vi "configwrite_ini.vi"() -> ()   [LabVIEW 2013]
uses:
  <vilib>/Utility/config.llb/Write Key (Double).vi
  <vilib>/Utility/config.llb/Write Key (String).vi
  <vilib>/Utility/config.llb/NI_LVConfig.lvlib
panel:
  out "error out":errorcluster caption="错误输出"
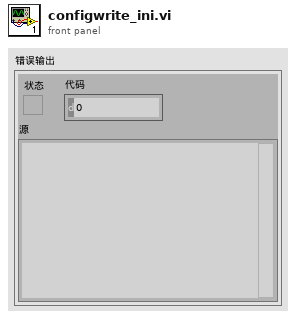
[diagram p1: front panel]
types:
  T1 = typedef "NI_LVConfig.lvlib/Config Data RefNum.ctl" = refnum<k1>
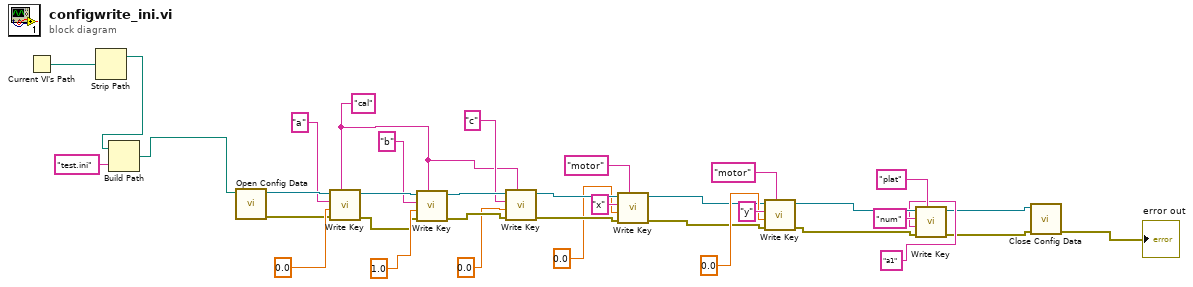
[diagram p0: block diagram]
diagram:
  w22 = "cal" ("section")
  n1 = Current VI's Path() -> (path=w2:path)
  n2 = Strip Path(path=w2) -> (stripped path=w1:path)  [unwired: 1 out]
  n3 = Build Path(base path=w1, name or relative path="test.ini" ("名称或相对路径")) -> (appended path=w3:path)
  n4 = call <vilib>:"Open Config Data.vi"("configuration file path"=w3) -> ("error out"=w27:errorcluster, "refnum"=w34:T1)  [unwired: 8 in, 1 out]
  n5 = call-poly <vilib>:"Write Key.vi"("section"=w22, "error in (no error)"=w27, "value"=0.0, "key"="a", "refnum"=w34) -> ("error out"=w28:errorcluster, "refnum out"=w31:T1)  [unwired: 4 in, 1 out]
  n6 = call-poly <vilib>:"Write Key.vi"("section"=w22, "error in (no error)"=w28, "value"=1.0, "key"="b", "refnum"=w31) -> ("error out"=w26:errorcluster, "refnum out"=w25:T1)  [unwired: 4 in, 1 out]
  n7 = call-poly <vilib>:"Write Key.vi"("section"=w22, "error in (no error)"=w26, "value"=0.0, "key"="c", "refnum"=w25) -> ("error out"=w21:errorcluster, "refnum out"=w20:T1)  [unwired: 4 in, 1 out]
  n8 = call-poly <vilib>:"Write Key.vi"("section"="motor", "error in (no error)"=w21, "value"=0.0, "key"="x", "refnum"=w20) -> ("error out"=w12:errorcluster, "refnum out"=w13:T1)  [unwired: 4 in, 1 out]
  n9 = call-poly <vilib>:"Write Key.vi"("section"="motor", "error in (no error)"=w12, "value"=0.0, "key"="y", "refnum"=w13) -> ("error out"=w8:errorcluster, "refnum out"=w9:T1)  [unwired: 4 in, 1 out]
  n10 = call-poly <vilib>:"Write Key.vi"("section"="plat", "error in (no error)"=w8, "value"="a1", "key"="num", "refnum"=w9) -> ("error out"=w6:errorcluster, "refnum out"=w5:T1)  [unwired: 4 in, 1 out]
  n11 = call <vilib>:"Close Config Data.vi"("error in (no error)"=w6, "refnum"=w5) -> ("error out"=→"error out":errorcluster)  [unwired: 8 in, 1 out]
